vi "Find Value.vi"(2 "Data":cluster{"Key":string, "Value":variant}[](array[cluster]), 3 "Key":string) -> (0 "Found":bool, 1 "Value":variant)   [LabVIEW 2018, in "Toolkit.lvlib" / "Render.lvclass"]
uses:
  Render.lvclass
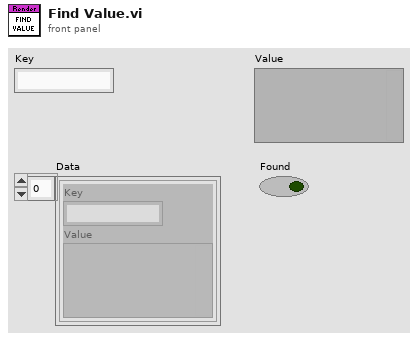
[diagram p1: front panel]
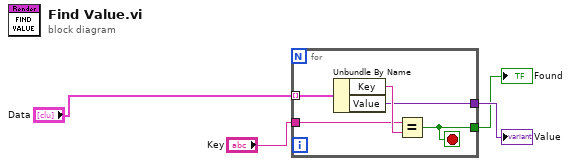
[diagram p0: block diagram]
diagram:
  n1 = for {
    tunnel: "Data" -> [w9] mode=indexing
    tunnel: "Key" -> [w7]
    tunnel: [w6] -> w2
    tunnel: [w5] -> w3
    stop <- w6 stop-if-true
    n2 = Unbundle By Name(w9) -> ("Key"=w8:string, "Value"=w5:variant)
    n3 = Equal?(x=w7, y=w8) -> (x = y?=w6:bool)
  }
  "Value" <- w3
  "Found" <- w2
